vi "RTP_RTSP - SETUP - METHOD.vi"(0 "RTSP Session":T1, 9 "timeout ms (1000)":i32=1000, 11 "error in (no error)":errorcluster) -> (4 "RTSP Session 2":T1, 15 "error out":errorcluster)   [LabVIEW 2014]
uses:
  RTSP Session.ctl
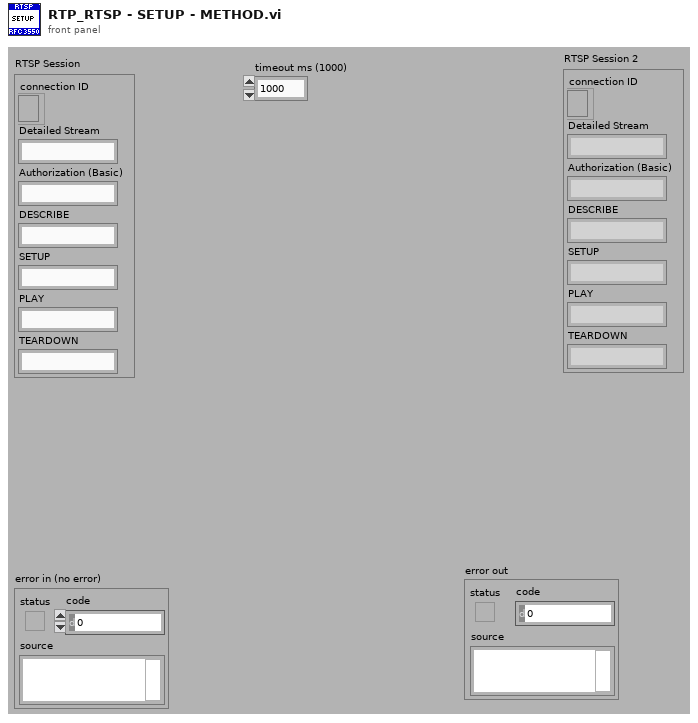
[diagram p1: front panel]
types:
  T1 = typedef "RTSP Session.ctl" = cluster{"connection ID":refnum<k5>, "Authorization (Basic)":string, "Detailed Stream":string, "DESCRIBE":string, "SETUP":string, "PLAY":string, "TEARDOWN":string}
  T2 = enum16{"Standard", "Buffered", "CRLF", "Immediate"}
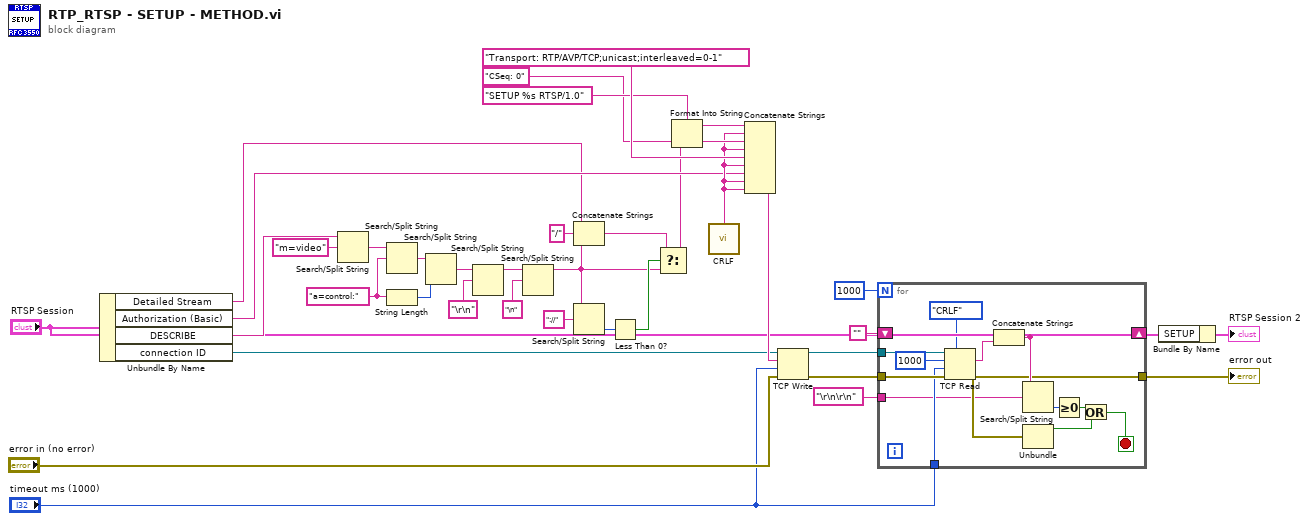
[diagram p0: block diagram]
diagram:
  w33 = "a=control:" ("search string/char (-)")
  n1 = Unbundle By Name("RTSP Session") -> ("Detailed Stream"=w5:string, "Authorization (Basic)"=w6:string, "DESCRIBE"=w7:string, "connection ID"=w8:refnum<k5>)
  n2 = Search/Split String(string=w7, search string/char (-)="m=video") -> (match + rest of string=w30:string)  [unwired: 1 in, 2 out]
  n3 = Search/Split String(string=w30, search string/char (-)=w33) -> (match + rest of string=w31:string)  [unwired: 1 in, 2 out]
  n4 = String Length(string=w33) -> (length=w32:i32)
  n5 = Search/Split String(string=w31, offset (0)=w32) -> (match + rest of string=w34:string)  [unwired: 1 in, 2 out]
  n6 = Search/Split String(string=w34, search string/char (-)="\r\n") -> (substring before match=w11:string)  [unwired: 1 in, 2 out]
  n7 = Search/Split String(string=w11, search string/char (-)="\n") -> (substring before match=w10:string)  [unwired: 1 in, 2 out]
  n8 = Concatenate Strings(w5, "/" ("string"), w10) -> (w21:string)
  n9 = Search/Split String(string=w10, search string/char (-)="://") -> (offset of match=w23:i32)  [unwired: 1 in, 2 out]
  n10 = Less Than 0?(x=w23) -> (x < 0?=w22:bool)
  n11 = Select(t=w21, s=w22, f=w10) -> (s? t:f=w1:string)
  n12 = Format Into String(format string="SETUP %s RTSP/1.0", w1) -> (resulting string=w27:string)  [unwired: 2 in, 1 out]
  n13 = call "CRLF.vi"() -> ("CRLF"=w20:string)
  n14 = Concatenate Strings(w27, w20, "CSeq: 0" ("string"), w20, "Transport: RTP/AVP/TCP;unicast;interleaved=0-1", w20, w6, w20, w20) -> (w26:string)
  n15 = TCP Write(connection ID=w8, data in=w26, error in (no error)="error in (no error)", 9:"timeout ms (1000)") -> (connection ID out=w17:refnum<k5>, error out=w16:errorcluster)  [unwired: 1 out]
  n16 = for {
    N: 1000 -> [_]
    tunnel: w16 -> [w51]
    tunnel: w17 -> [w50]
    tunnel: [w42] -> w13
    shift-right: [w44] -> w2
    shift-left: "" -> [w48]
    tunnel: "timeout ms (1000)" -> [w45]
    tunnel: "\r\n\r\n" ("search string/char (-)") -> [w41]
    stop <- w38 stop-if-true
    n17 = TCP Read(connection ID=w50, bytes to read=1000, error in (no error)=w51, 7:T2."CRLF" ("mode (standard)"), 9:w45) -> (data out=w47:string, error out=w42:errorcluster)  [unwired: 1 out]
    n18 = Concatenate Strings(w48, w47) -> (w44:string)
    n19 = Search/Split String(string=w44, search string/char (-)=w41) -> (offset of match=w43:i32)  [unwired: 1 in, 2 out]
    n20 = Unbundle(w42) -> ("status"=w39:bool)  [unwired: 2 out]
    n21 = Greater Or Equal To 0?(x=w43) -> (x >= 0?=w40:bool)
    n22 = Or(x=w40, y=w39) -> (x .or. y?=w38:bool)
  }
  "error out" <- w13
  n23 = Bundle By Name(cluster="RTSP Session", "SETUP"=w2) -> (→"RTSP Session 2":T1)
